vi "close_tcp_connections.vi"(4 "error in":errorcluster) -> (0 "error out":errorcluster)   [LabVIEW 2019, in "Lib_Simx.lvlib"]
doc: "Close all the TCP references opened by the client."
uses:
  Lib_Simx.lvlib
  tools/simx_common.vi
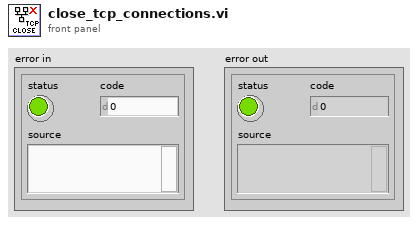
[diagram p1: front panel]
types:
  T1 = typedef "Lib_Simx.lvlib/simx_connection.ctl" = cluster{"Config":T2, "Connections":T5, "Map":cluster{"lanes":cluster{"x":dbl[], "y":dbl[], "z":dbl[]}, "StartPosition":cluster{"start_points":T6, "StartRotation":dbl[], "StartLocation":dbl[]}, "Draw Map Size":T7, "DrawArea":cluster{"min_Y":dbl, "min_X":dbl, "Scale X":dbl, "Scale Y":dbl}, "Map":picture, "Map Geojson":string}}
  T2 = typedef "Lib_Simx.lvlib/config.ctl" = cluster{"Trajectory":T3, "Weather":T4}
  T3 = typedef "Lib_Simx.lvlib/trajectory.ctl" = cluster{"Number of frames":i32, "Frame number":i32, "Trajectory":string}
  T4 = typedef "Lib_Simx.lvlib/weather.ctl" = cluster{"id":string}
  T5 = typedef "Lib_Simx.lvlib/connections.ctl" = cluster{"Simulator Connection":refnum<k5>, "server_ip":string, "Port":i32, "Sensor connections":refnum<k5>[]}
  T6 = typedef "Lib_Simx.lvlib/start_points.ctl" = cluster{"locations":dbl[][], "rotations":dbl[][], "type":string[]}
  T7 = typedef "LVBoundsTypeDef.ctl" = cluster{"Width":u32, "Height":u32}
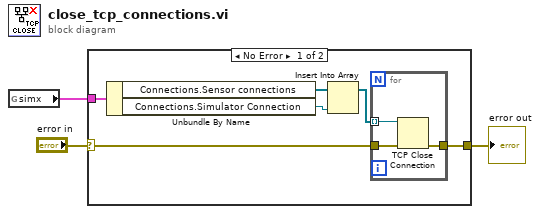
[diagram p0: block diagram]
diagram:
  n1 = global read "simx_common.vi" "simx"() -> (w2:T1)
  n2 = case shown="No Error" "error in" {
    selector: "error in" -> [w4 w13]
    tunnel: [w9 w13] -> w3
    tunnel: w2 -> [w7 _]
    frame No Error {
      n3 = Unbundle By Name(w7) -> ("Connections.Sensor connections"=w8:refnum<k5>[], "Connections.Simulator Connection"=w5:refnum<k5>)
      n4 = Insert Into Array(array=w8, new element=w5) -> (w6:refnum<k5>[])  [unwired: 1 in]
      n5 = for {
        tunnel: w6 -> [w12] mode=indexing
        tunnel: w4 -> [w11]
        tunnel: [w10] -> w9
        n6 = TCP Close Connection(connection ID=w12, error in (no error)=w11) -> (error out=w10:errorcluster)  [unwired: 1 in, 1 out]
      }
    }
    frame Error {
    }
  }
  "error out" <- w3
